vi "Report Export.vi"(4 "delimiter (\\t)":string="\t", 5 "Condition":bool, 7 "error in (no error)":errorcluster, 8 "Data":string[][](array[string]), 10 "Report Type":string) -> (0 "error out":errorcluster)   [LabVIEW 2024]
uses:
  <vilib>/Utility/file.llb/Write Delimited Spreadsheet (string).vi
panel:
  out "selected path":path
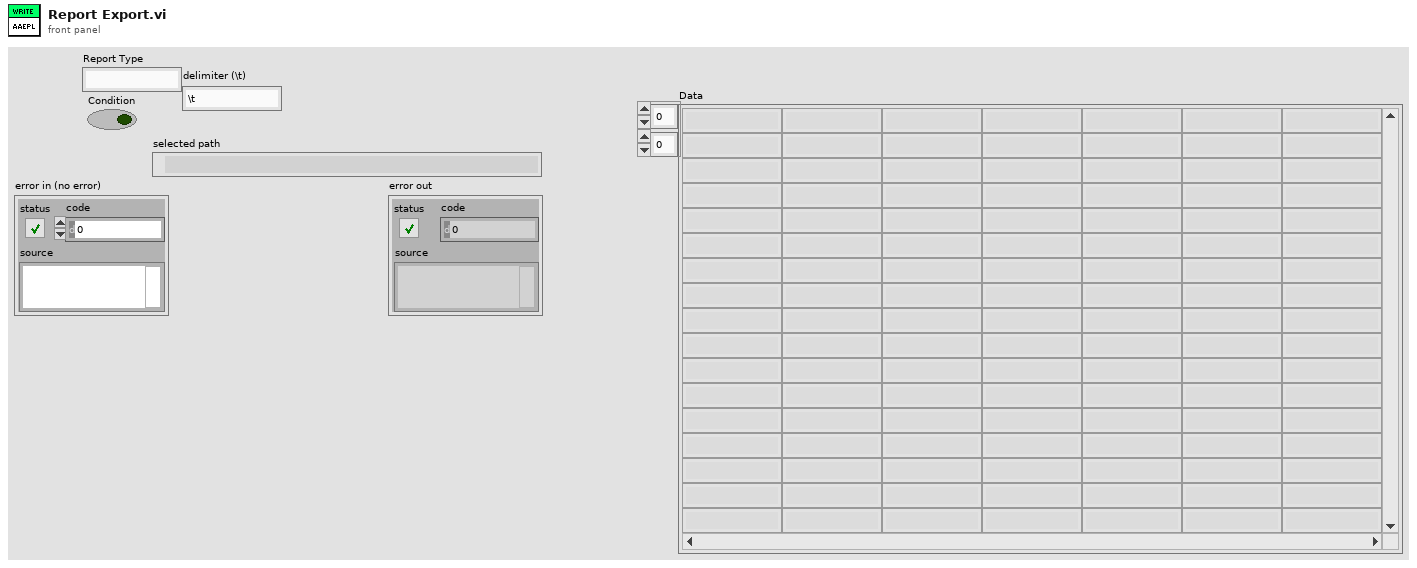
[diagram p1: front panel]
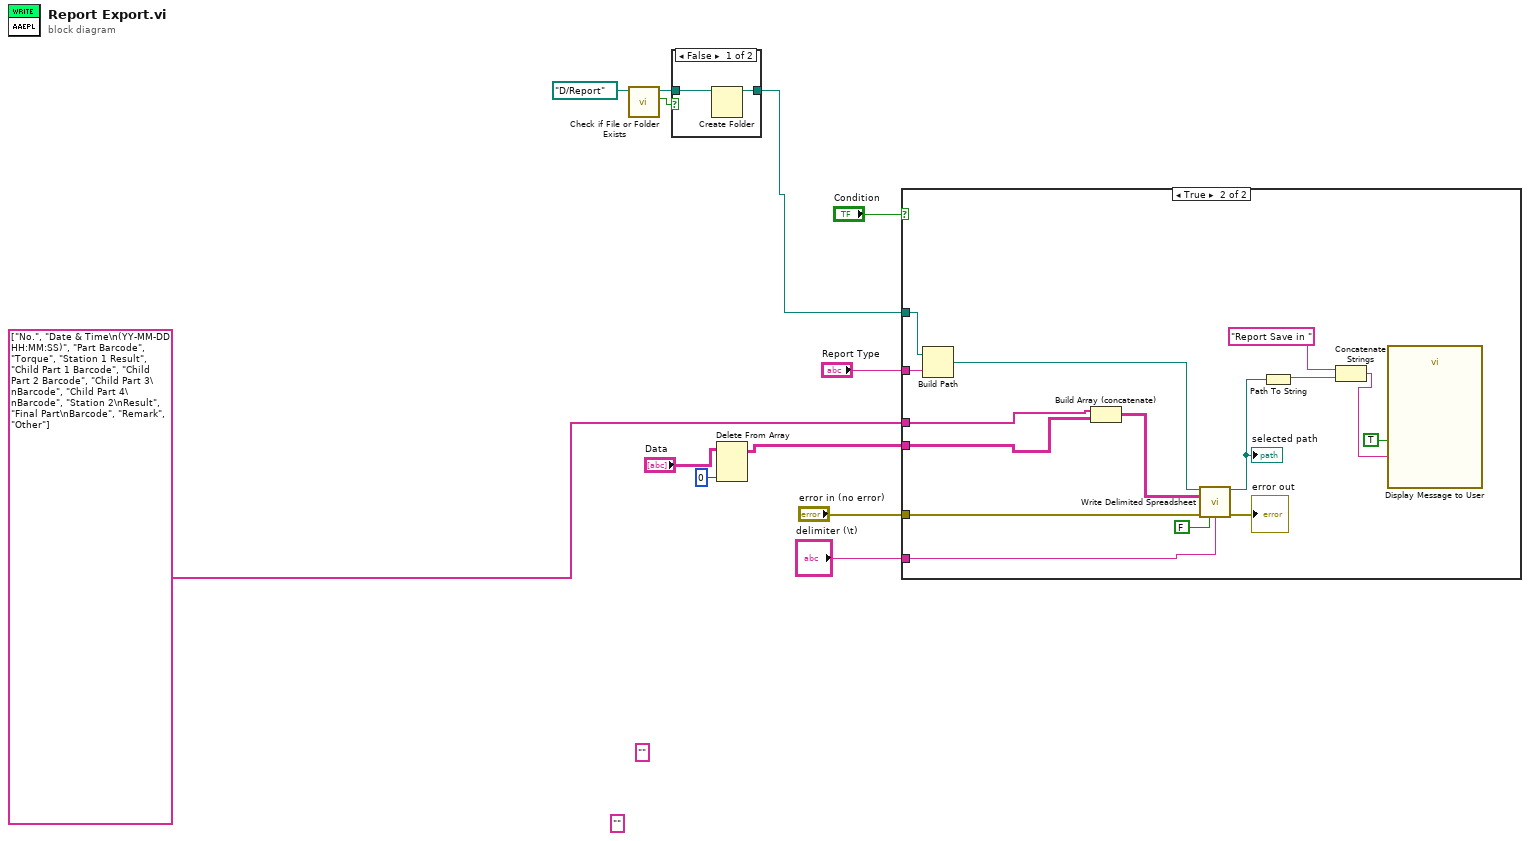
[diagram p0: block diagram]
diagram:
  (unwired) ""
  (unwired) ""
  n1 = call <vilib>:"Check if File or Folder Exists.vi"("path"=path "D:/Report" ("selected path 2")) -> ("file or folder exists?"=w7:bool, "dup path"=w6:path)  [unwired: 8 in, 1 out]
  n2 = case shown="False" w7 {
    tunnel: w6 -> [w14 w15]
    tunnel: [w13 w15] -> w5
    frame False {
      n3 = Create Folder(path (use dialog)=w14) -> (created path=w13:path)  [unwired: 2 in, 2 out]
    }
    frame True {
    }
  }
  n4 = Delete From Array(array="Data", index (col)=0 ("disabled index (col)")) -> (array with subset deleted=w3:string[][])  [unwired: 2 in, 1 out]
  n5 = case shown="True" "Condition" {
    tunnel: w5 -> [_ w30]
    tunnel: "Report Type" -> [_ w29]
    tunnel: "error in (no error)" -> [_ w28]
    tunnel: w3 -> [_ w27]
    tunnel: "delimiter (\\t)" -> [_ w22]
    tunnel: string[] ["No.", "Date & Time\n(YY-MM-DD HH:MM:SS)", "Part Barcode", "Torque", "Station 1 Result", "Child Part 1 Barcode", "Child Part 2 Barcode", "Child Part 3\nBarcode", "Child Part 4\nBarcode", "Station 2\nResult", "Final Part\nBarcode", "Remark", "Other"] ("Column Header Strings[]") -> [_ w21]
    frame False {
    }
    frame True {
      n6 = Build Path(base path=w30, name or relative path=w29) -> (appended path=w25:path)
      n7 = Build Array (concatenate)(w21, w27) -> (w26:string[][])
      n8 = call-poly <vilib>:"Write Delimited Spreadsheet.vi"("file path (dialog if empty)"=w25, "2D data"=w26, "error in (no error)"=w28, "transpose? (no:F)"=FALSE ("transpose? (F)"), "delimiter (\\t)"=w22) -> ("new file path (Not A Path if cancelled)"=w19:path, "error out"=→"error out":errorcluster)  [unwired: 9 in]
      "selected path" <- w19
      n9 = Path To String(path=w19) -> (string=w17:string)
      n10 = Concatenate Strings("Report Save in " ("string"), w17) -> (w16:string)
      n11 = call "Display Message to User"("Enable"=TRUE, "Message"=w16) -> ()  [unwired: 8 in, 2 out]
    }
  }
